vi "Read ADC.vi"(8 "error in (no error)":errorcluster, 11 "NAU7802 in":refnum<class "Adafruit NAU7802 24bit Strain Gauge.lvclass">) -> (0 "error out":errorcluster, 2 "Data Out":dbl, 3 "NAU7802 out":refnum<class "Adafruit NAU7802 24bit Strain Gauge.lvclass">)   [LabVIEW 2020, in "CTI-Peripheral.lvlib" / "Adafruit NAU7802 24bit Strain Gauge.lvclass"]
uses:
  Adafruit NAU7802 24bit Strain Gauge.lvclass
  Adafruit NAU7802 24bit Strain Gauge.lvclass/Adafruit NAU7802 24bit Strain Gauge.ctl
  CTI/I2C Connection/I2C Connection.lvclass/I2C Connection.ctl
  CTI/Session/I2C Write Data.vi
  CTI/Session/I2C Read Data.vi
  CTI/I2C Connection/I2C Connection.lvclass
panel:
  out "Data":string
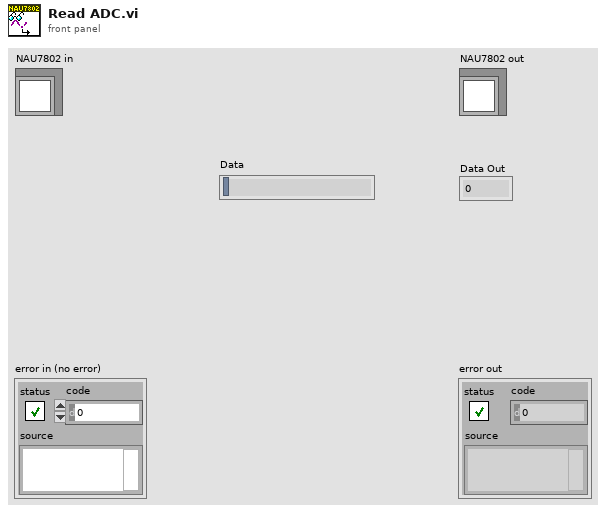
[diagram p1: front panel]
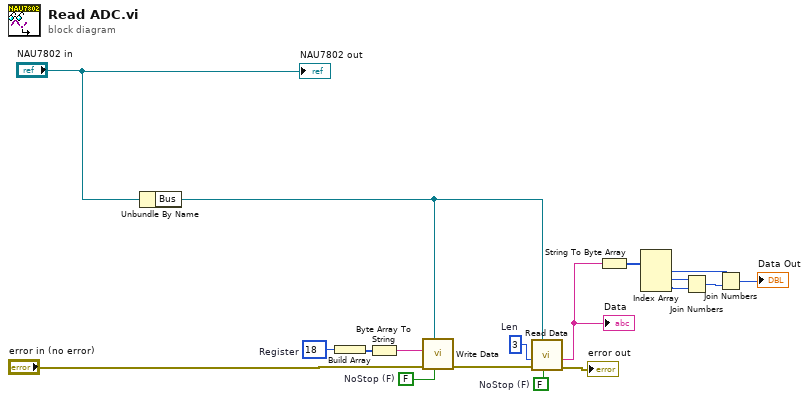
[diagram p0: block diagram]
diagram:
  w6 = u8 18  # Register
  w14 = FALSE  # NoStop (F)
  w15 = u8 3  # Len
  w16 = FALSE  # NoStop (F)
  n1 = Unbundle By Name("NAU7802 in") -> ("Bus"=w13:refnum<class "I2C Connection.lvclass">)
  n2 = Build Array(w6) -> (w7:u8[])
  n3 = Byte Array To String(unsigned byte array=w7) -> (string=w5:string)
  n4 = call "Write Data.vi"("NoStop (F)"=w16, "I2C Connection"=w13, "error in (no error)"="error in (no error)", "Data"=w5) -> ("error out"=w12:errorcluster)  [unwired: 7 in]
  n5 = call "Read Data.vi"("NoStop (F)"=w14, "I2C Connection"=w13, "error in (no error)"=w12, "Len"=w15) -> ("error out"=→"error out":errorcluster, "Data"=w4:string)  [unwired: 6 in]
  "Data" <- w4
  n6 = String To Byte Array(string=w4) -> (unsigned byte array=w10:u8[])
  n7 = Index Array(array=w10) -> (element #1=w1:u8, element #2=w9:u8, element #3=w8:u8)  [unwired: 3 in]
  n8 = Join Numbers(hi=w9, lo=w8) -> ((hi.lo)=w2:u16)
  n9 = Join Numbers(hi=w1, lo=w2) -> ((hi.lo)=→"Data Out":u32)
  "NAU7802 out" <- "NAU7802 in"
